vi "Autonomous Independent.vi"() -> ()   [LabVIEW 2014]
doc: "This VI is called when autonomous begins, and will automatically be terminated when autonomous ends. You can carry out timed or sensor driven robot movement independently without needing to return to the caller."
uses:
  <vilib>/Rock Robotics/WPI/Joystick/WPI_JoystickGetSetRefNum.vi
  <vilib>/Rock Robotics/Network Tables/SD Read Boolean.vi
  <vilib>/Rock Robotics/WPI/RobotDrive/WPI_RobotDriveGetSetRefNum.vi
  <vilib>/Rock Robotics/WPI/RobotDrive/WPI_RobotDriveArcadeDrive_Standard(NoSaturation).vi
  <vilib>/Rock Robotics/Network Tables/SD Write Boolean.vi
panel:
  out "Sample Boolean 2":bool
  out "Sample Boolean 3":bool
  out "Sample Boolean 1":bool
  out "Sample Boolean 0":bool
  out "Current Movement, for debugging":T1 {"Y Joystick Value" scale=1.0..-1.0; "X Joystick Value" scale=-1.0..1.0}
  in  "Array of robot movements":T2(array[cluster]) {"Y Joystick Value" scale=1.0..-1.0; "X Joystick Value" scale=-1.0..1.0}
  # "Be sure to right-click and choose Data Operations>>Make Current Value default if you want to save the array values with the VI"
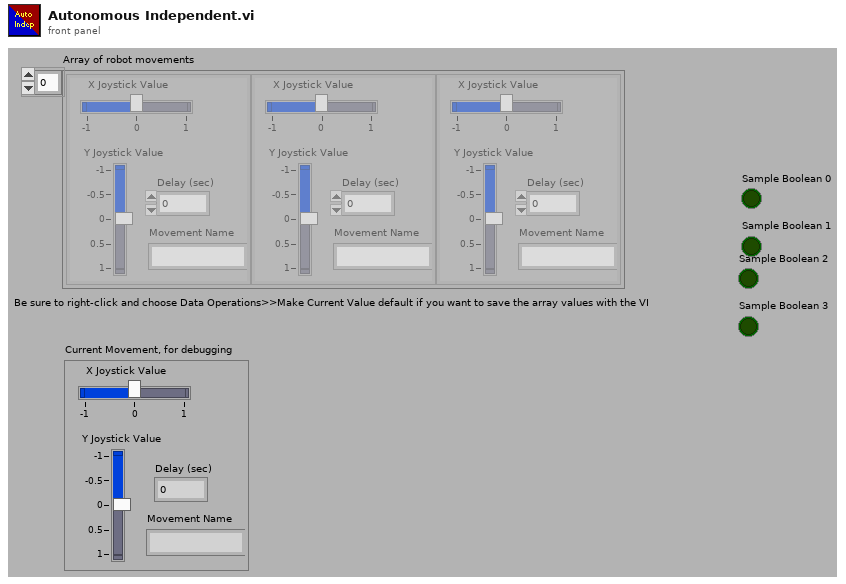
[diagram p1: front panel]
types:
  T1 = cluster{"X Joystick Value":dbl, "Y Joystick Value":dbl, "Delay (sec)":dbl, "Movement Name":string}
  T2 = cluster{"X Joystick Value":dbl, "Y Joystick Value":dbl, "Delay (sec)":dbl, "Movement Name":string}[]
  T3 = typedef "WPI_JoystickDevRef.ctl" = cluster{"Device":T4}
  T4 = typedef "WPI_JoystickDeviceEnum.ctl" = enum16{"USB 0", "USB 1", "USB 2", "USB 3", "USB 4", "USB 5"}
  T5 = typedef "WPI_RobotDriveDevRef.ctl" = cluster{"DevStatus":errorcluster, "Motors[]":T6[], "Square Inputs":bool, "Max Output":dbl}
  T6 = typedef "WPI_MotorControlDeviceRef.ctl" = cluster{"DeviceStatus":errorcluster, "Type":T7, "PWM":cluster{"Controller":T8, "PWM Channel":T9, "DeadBand":T10}, "CAN":cluster{"Device Number":u8, "Control Mode":T11, "Semaphore":T12, "Max Vout":dbl, "TalonSRX Control Mode":T13}, "Invert":bool, "TransformRef":T14, "InvTransformRef":T14}
  T7 = typedef "WPI_MotorControlType.ctl" = enum16{"PWM", "CAN", "CANTalonSRX"}
  T8 = typedef "FPGA_TypedefDigitalModule.ctl" = enum16{"Controller 1"}
  T9 = typedef "FPGA_DIOPWMChannel.ctl" = enum8{"PWM 0", "PWM 1", "PWM 2", "PWM 3", "PWM 4", "PWM 5", "PWM 6", "PWM 7", "PWM 8", "PWM 9", "PWM MXP 0", "PWM MXP 1", "PWM MXP 2", "PWM MXP 3", "PWM MXP 4", "PWM MXP 5", "PWM MXP 6", "PWM MXP 7", "PWM MXP 8", "PWM MXP 9", "Invalid"}
  T10 = typedef "WPI_PWMDeadband.ctl" = cluster{"Name":string, "maxPositivePwm":i32, "minPositivePwm":i32, "centerPwm":i32, "maxNegativePwm":i32, "minNegativePwm":i32, "angularRange":u16}
  T11 = typedef "WPI_CANJaguar_ControlMode.ctl" = enum8{"Percent VBus", "Current", "Speed", "Position", "Voltage"}
  T12 = typedef "Semaphore RefNum" = refnum<k1>
  T13 = typedef "WPI_CANTalonSRX_APIControlMode.ctl" = enum8{"Percent VBus", "Speed", "Position", "Slave", "Unchanged / Invalid"}
  T14 = typedef "WPI_PWMTransform_ConPane.ctl" = refnum<vi>
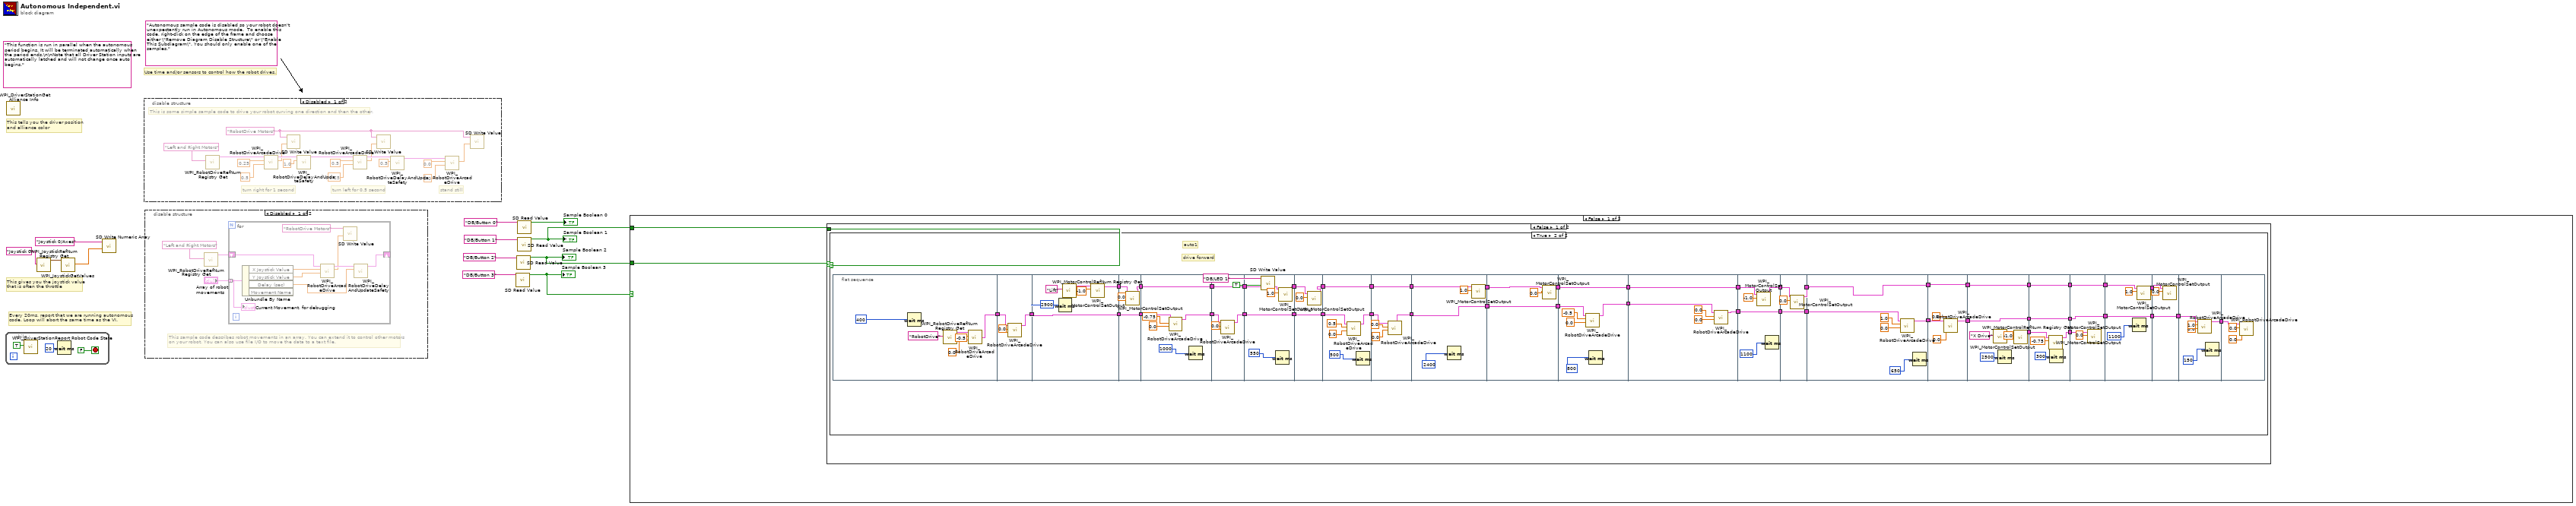
[diagram p0: block diagram]
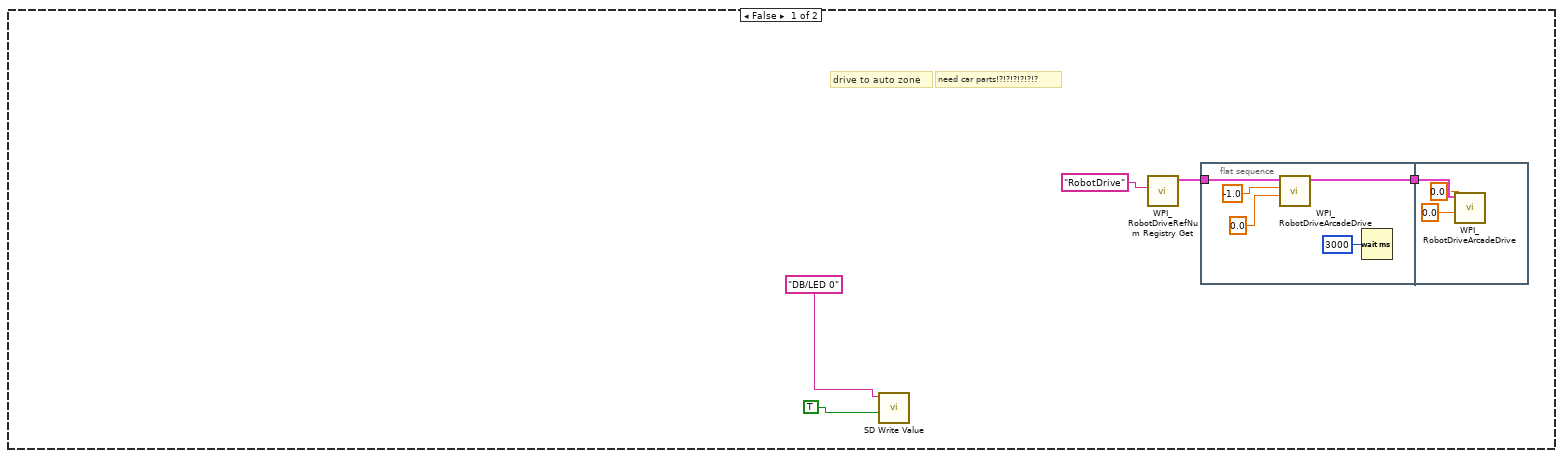
[diagram p2: hidden frame]
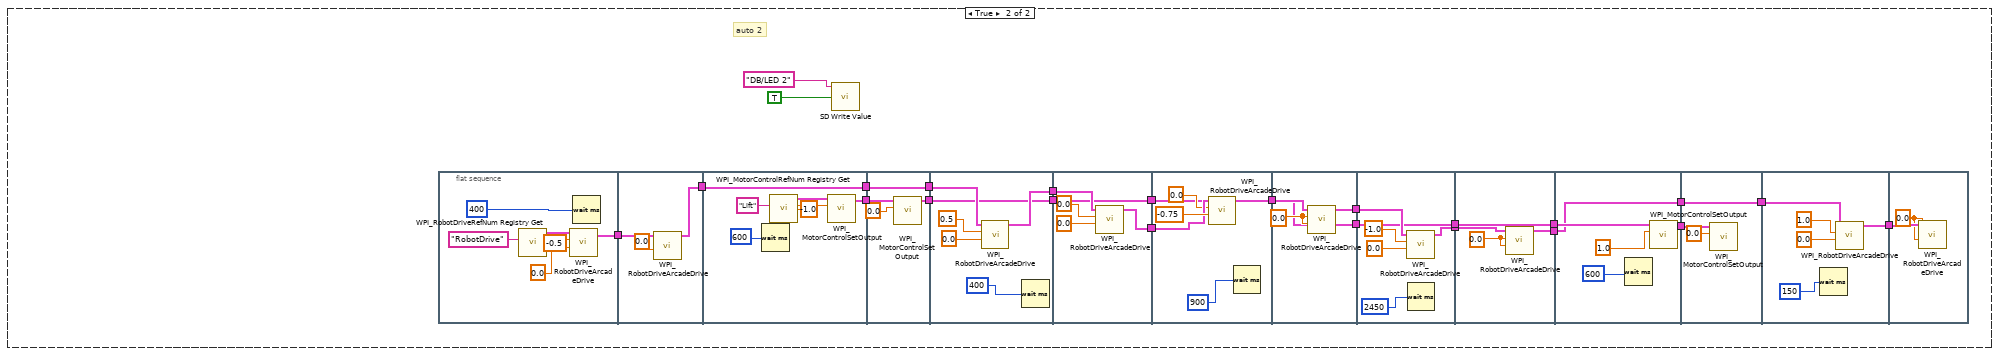
[diagram p3: hidden frame]
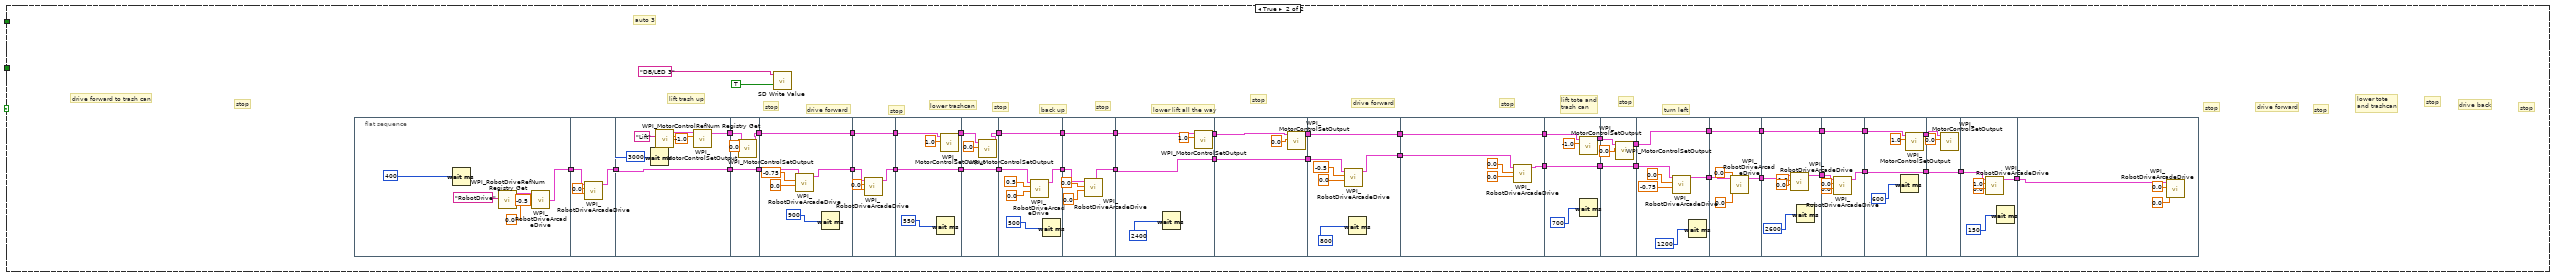
[diagram p4: hidden frame]
diagram:
  (unwired) "Autonomous sample code is disabled so your robot doesn't unexpectantly run in Autonomous mode.  To enable this code, right-click on the edge of the frame and choose either \"Remove Diagram Disable Structure\" or \"Enable This Subdiagram\". You should only enable one of the samples."
  (unwired) "This function is run in parallel when the autonomous period begins. It will be terminated automatically when the period ends.\n\nNote that all Driver Station inputs are automatically latched and will not change once auto begins."
  # "Every 20ms, report that we are running autonomous\ncode. Loop will abort the same time as the VI."
  # "This gives you the joystick value\nthat is often the throttle"
  # "Use time and/or sensors to control how the robot drives."
  # "This tells you the driver position\nand alliance color"
  n1 = while {
    stop <- FALSE stop-if-true
    n2 = call <vilib>:"WPI_DriverStationReport Robot Code State.vi"("Autonomous"=TRUE) -> ()  [unwired: 10 in, 1 out]
    n3 = Wait (ms)(milliseconds to wait=u32 20) -> ()  [unwired: 1 out]
  }
  n4 = call <vilib>:"WPI_DriverStationGet Alliance Info.vi"() -> ()  [unwired: 12 out]
  n5 = call <vilib>:"WPI_JoystickRefNum Registry Get.vi"("refnum name"="Joystick 0") -> ("JoystickDevRef"=w11:T3)  [unwired: 1 in, 9 out]
  n6 = call <vilib>:"WPI_JoystickGetValues.vi"("JoystickDevRef"=w11) -> ("Axes"=w9:dbl[])  [unwired: 6 in, 4 out]
  n7 = call <vilib>:"SD Write Numeric Array.vi"("Numeric Array"=w9, "Name"="Joystick 0/Axes") -> ()  [unwired: 8 in, 2 out]
  n8 = disable-structure shown="Disabled" {
    frame Disabled {
      w19 = "RobotDrive Motors" ("Name")
      # "This is some simple sample code to drive your robot curving one direction and then the other."
      # "stand still"
      # "turn left for 0.5 second"
      # "turn right for 1 second"
      n9 = call <vilib>:"WPI_RobotDriveRefNum Registry Get.vi"("refnum name"="Left and Right Motors") -> ("RobotDriveDevRef"=w20:T5)  [unwired: 1 in, 9 out]
      n10 = call-poly <vilib>:"WPI_RobotDriveArcadeDrive.vi"("Y axis value"=0.5 ("X axis value"), "X axis value"=0.25, "RobotDriveDevRef"=w20) -> ("Motor Values"=w18:dbl[], "RobotDriveDevRef"=w27:T5)  [unwired: 1 in, 6 out]
      n11 = call-poly <vilib>:"SD Write Value.vi"("Numeric Array"=w18, "Name"=w19) -> ()  [unwired: 8 in, 2 out]
      n12 = call <vilib>:"WPI_RobotDriveDelayAndUpdateSafety.vi"("Delay (s)"=1.0, "RobotDriveDevRef"=w27) -> ("RobotDriveDevRef 2"=w26:T5)  [unwired: 8 in, 1 out]
      n13 = call-poly <vilib>:"WPI_RobotDriveArcadeDrive.vi"("Y axis value"=0.25 ("X axis value"), "X axis value"=0.5, "RobotDriveDevRef"=w26) -> ("Motor Values"=w17:dbl[], "RobotDriveDevRef"=w25:T5)  [unwired: 1 in, 6 out]
      n14 = call-poly <vilib>:"SD Write Value.vi"("Numeric Array"=w17, "Name"=w19) -> ()  [unwired: 8 in, 2 out]
      n15 = call <vilib>:"WPI_RobotDriveDelayAndUpdateSafety.vi"("Delay (s)"=0.5, "RobotDriveDevRef"=w25) -> ("RobotDriveDevRef 2"=w24:T5)  [unwired: 8 in, 1 out]
      n16 = call-poly <vilib>:"WPI_RobotDriveArcadeDrive.vi"("Y axis value"=0.0 ("X axis value"), "X axis value"=0.0, "RobotDriveDevRef"=w24) -> ("Motor Values"=w16:dbl[])  [unwired: 1 in, 7 out]
      n17 = call-poly <vilib>:"SD Write Value.vi"("Numeric Array"=w16, "Name"=w19) -> ()  [unwired: 8 in, 2 out]
    }
    frame Enabled {
    }
  }
  n18 = disable-structure shown="Disabled" {
    frame Disabled {
      # "This sample code describes robot movements in an array. You can extend it to control other motors\non your robot. You can also use file I/O to move the data to a text file."
      n19 = call <vilib>:"WPI_RobotDriveRefNum Registry Get.vi"("refnum name"="Left and Right Motors") -> ("RobotDriveDevRef"=w35:T5)  [unwired: 1 in, 9 out]
      n20 = for {
        shift-right: [w42] -> _
        shift-left: w35 -> [w43]
        tunnel: "Array of robot movements" -> [w38] mode=indexing
        n21 = Unbundle By Name(w38) -> ("X Joystick Value"=w41:dbl, "Y Joystick Value"=w40:dbl, "Delay (sec)"=w39:dbl)  [unwired: 1 out]
        n22 = call-poly <vilib>:"WPI_RobotDriveArcadeDrive.vi"("Y axis value"=w40, "X axis value"=w41, "RobotDriveDevRef"=w43) -> ("Motor Values"=w37:dbl[], "RobotDriveDevRef"=w44:T5)  [unwired: 1 in, 6 out]
        n23 = call-poly <vilib>:"SD Write Value.vi"("Numeric Array"=w37, "Name"="RobotDrive Motors") -> ()  [unwired: 8 in, 2 out]
        n24 = call <vilib>:"WPI_RobotDriveDelayAndUpdateSafety.vi"("Delay (s)"=w39, "RobotDriveDevRef"=w44) -> ("RobotDriveDevRef 2"=w42:T5)  [unwired: 8 in, 1 out]
        "Current Movement, for debugging" <- w38
      }
    }
    frame Enabled {
    }
  }
  n25 = call-poly <vilib>:"SD Read Value.vi"("Name"="DB/Button 3" ("refnum name")) -> ("Boolean"=w3:bool)  [unwired: 8 in, 2 out]
  "Sample Boolean 3" <- w3
  n26 = call-poly <vilib>:"SD Read Value.vi"("Name"="DB/Button 2" ("refnum name")) -> ("Boolean"=w2:bool)  [unwired: 8 in, 2 out]
  "Sample Boolean 2" <- w2
  n27 = call-poly <vilib>:"SD Read Value.vi"("Name"="DB/Button 1" ("refnum name")) -> ("Boolean"=w1:bool)  [unwired: 8 in, 2 out]
  "Sample Boolean 1" <- w1
  n28 = call-poly <vilib>:"SD Read Value.vi"("Name"="DB/Button 0" ("refnum name")) -> ("Boolean"=→"Sample Boolean 0":bool)  [unwired: 8 in, 2 out]
  n29 = case shown="False" w3 {
    tunnel: w2 -> [w47 _]
    tunnel: w1 -> [w46 _]
    frame False {
      n30 = case shown="False" w47 {
        tunnel: w46 -> [w48 _]
        frame False {
          n31 = case shown="True" w48 {
            frame False {
              # "need car parts!?!?!?!?!?!?"
              # "drive to auto zone"
              n32 = call-poly <vilib>:"SD Write Value.vi"("Boolean"=TRUE, "Name"="DB/LED 0" ("refnum name")) -> ()  [unwired: 8 in, 2 out]
              n33 = call <vilib>:"WPI_RobotDriveRefNum Registry Get.vi"("refnum name"="RobotDrive") -> ("RobotDriveDevRef"=w53:T5)  [unwired: 1 in, 9 out]
              n34 = flat-sequence {
                tunnel: w53 -> [w56]
                tunnel: [w54] -> w49
                tunnel: w49 -> [w61]
                frame #0 {
                  n35 = call-poly <vilib>:"WPI_RobotDriveArcadeDrive.vi"("Y axis value"=0.0 ("X axis value"), "X axis value"=-1.0, "RobotDriveDevRef"=w56) -> ("RobotDriveDevRef"=w54:T5)  [unwired: 1 in, 7 out]
                  n36 = Wait (ms)(milliseconds to wait=u32 3000) -> ()  [unwired: 1 out]
                }
                frame #1 {
                  n37 = call-poly <vilib>:"WPI_RobotDriveArcadeDrive.vi"("Y axis value"=0.0, "X axis value"=0.0, "RobotDriveDevRef"=w61) -> ()  [unwired: 1 in, 8 out]
                }
              }
            }
            frame True {
              # "drive forward"
              # "auto1"
              n38 = flat-sequence {
                tunnel: [w111] -> w107
                tunnel: w107 -> [w118]
                tunnel: [w117] -> w106
                tunnel: w106 -> [w121]
                tunnel: [w121] -> w105
                tunnel: [w119] -> w104
                tunnel: w105 -> [w128]
                tunnel: [w128] -> w103
                tunnel: w104 -> [w127]
                tunnel: [w126] -> w102
                tunnel: w103 -> [w132]
                tunnel: [w131] -> w101
                tunnel: w102 -> [w129]
                tunnel: [w129] -> w100
                tunnel: w101 -> [w137]
                tunnel: [w136] -> w99
                tunnel: w100 -> [w138]
                tunnel: [w138] -> w98
                tunnel: w99 -> [w143]
                tunnel: [w143] -> w97
                tunnel: w98 -> [w141]
                tunnel: [w140] -> w96
                tunnel: w97 -> [w147]
                tunnel: [w147] -> w95
                tunnel: w96 -> [w145]
                tunnel: [w144] -> w94
                tunnel: w95 -> [w152]
                tunnel: [w151] -> w93
                tunnel: w94 -> [w153]
                tunnel: [w153] -> w92
                tunnel: w93 -> [w157]
                tunnel: [w156] -> w91
                tunnel: w92 -> [w158]
                tunnel: [w158] -> w90
                tunnel: w91 -> [w162]
                tunnel: [w162] -> w89
                tunnel: [w161] -> w88
                tunnel: w90 -> [w160]
                tunnel: w89 -> [w167]
                tunnel: [w167] -> w87
                tunnel: w88 -> [w165]
                tunnel: [w164] -> w86
                tunnel: w87 -> [w171]
                tunnel: [w170] -> w85
                tunnel: w86 -> [w168]
                tunnel: [w168] -> w84
                tunnel: w85 -> [w176]
                tunnel: w84 -> [w175]
                tunnel: [w175] -> w73
                tunnel: [w174] -> w72
                tunnel: w73 -> [w181]
                tunnel: [w180] -> w71
                tunnel: w72 -> [w183]
                tunnel: [w183] -> w69
                tunnel: w71 -> [w186]
                tunnel: [w185] -> w70
                tunnel: w69 -> [w187]
                tunnel: [w187] -> w68
                tunnel: [w189] -> w83
                tunnel: [w188] -> w82
                tunnel: w70 -> [w188]
                tunnel: w68 -> [w191]
                tunnel: w83 -> [w198]
                tunnel: [w195] -> w81
                tunnel: w82 -> [w194]
                tunnel: [w194] -> w80
                tunnel: w81 -> [w204]
                tunnel: w80 -> [w205]
                tunnel: [w205] -> w67
                tunnel: [w204] -> w65
                tunnel: [w200] -> w63
                tunnel: w67 -> [w211]
                tunnel: [w211] -> w66
                tunnel: w65 -> [w210]
                tunnel: [w210] -> w64
                tunnel: w63 -> [w208]
                tunnel: [w209] -> w62
                tunnel: w66 -> [w215]
                tunnel: [w215] -> w79
                tunnel: [w214] -> w78
                tunnel: w64 -> [w214]
                tunnel: w62 -> [w213]
                tunnel: [w219] -> w77
                tunnel: w79 -> [w218]
                tunnel: [w216] -> w76
                tunnel: w78 -> [w216]
                tunnel: w77 -> [w222]
                tunnel: [w221] -> w75
                tunnel: w76 -> [w221]
                tunnel: w75 -> [w228]
                tunnel: [w224] -> w74
                tunnel: w74 -> [w231]
                frame #0 {
                  n39 = Wait (ms)(milliseconds to wait=u32 400) -> ()  [unwired: 1 out]
                  n40 = call <vilib>:"WPI_RobotDriveRefNum Registry Get.vi"("refnum name"="RobotDrive") -> ("RobotDriveDevRef"=w114:T5)  [unwired: 1 in, 9 out]
                  n41 = call-poly <vilib>:"WPI_RobotDriveArcadeDrive.vi"("Y axis value"=0.0 ("X axis value"), "X axis value"=-0.5, "RobotDriveDevRef"=w114) -> ("RobotDriveDevRef"=w111:T5)  [unwired: 1 in, 7 out]
                }
                frame #1 {
                  w116 = 0.0 ("X axis value")
                  n42 = call-poly <vilib>:"WPI_RobotDriveArcadeDrive.vi"("Y axis value"=w116, "X axis value"=w116, "RobotDriveDevRef"=w118) -> ("RobotDriveDevRef"=w117:T5)  [unwired: 1 in, 7 out]
                }
                frame #2 {
                  n43 = Wait (ms)(milliseconds to wait=u32 2900) -> ()  [unwired: 1 out]
                  n44 = call <vilib>:"WPI_MotorControlRefNum Registry Get.vi"("refnum name"="Lift") -> ("MotorControlDevRef"=w123:T6)  [unwired: 9 in, 1 out]
                  n45 = call <vilib>:"WPI_MotorControlSetOutput.vi"("Output"=-1.0, "MotorControlDevRef"=w123) -> ("MotorControlDevRef"=w119:T6)  [unwired: 7 in, 2 out]
                }
                frame #3 {
                  n46 = call <vilib>:"WPI_MotorControlSetOutput.vi"("Output"=0.0, "MotorControlDevRef"=w127) -> ("MotorControlDevRef"=w126:T6)  [unwired: 7 in, 2 out]
                }
                frame #4 {
                  n47 = call-poly <vilib>:"WPI_RobotDriveArcadeDrive.vi"("Y axis value"=0.0 ("X axis value"), "X axis value"=-0.75, "RobotDriveDevRef"=w132) -> ("RobotDriveDevRef"=w131:T5)  [unwired: 1 in, 7 out]
                  n48 = Wait (ms)(milliseconds to wait=u32 1000) -> ()  [unwired: 1 out]
                }
                frame #5 {
                  w135 = 0.0 ("X axis value")
                  n49 = call-poly <vilib>:"WPI_RobotDriveArcadeDrive.vi"("Y axis value"=w135, "X axis value"=w135, "RobotDriveDevRef"=w137) -> ("RobotDriveDevRef"=w136:T5)  [unwired: 1 in, 7 out]
                }
                frame #6 {
                  n50 = Wait (ms)(milliseconds to wait=u32 550) -> ()  [unwired: 1 out]
                  n51 = call <vilib>:"WPI_MotorControlSetOutput.vi"("Output"=1.0, "MotorControlDevRef"=w141) -> ("MotorControlDevRef"=w140:T6)  [unwired: 7 in, 2 out]
                }
                frame #7 {
                  n52 = call <vilib>:"WPI_MotorControlSetOutput.vi"("Output"=0.0, "MotorControlDevRef"=w145) -> ("MotorControlDevRef"=w144:T6)  [unwired: 7 in, 2 out]
                }
                frame #8 {
                  n53 = call-poly <vilib>:"WPI_RobotDriveArcadeDrive.vi"("Y axis value"=0.0, "X axis value"=0.5, "RobotDriveDevRef"=w152) -> ("RobotDriveDevRef"=w151:T5)  [unwired: 1 in, 7 out]
                  n54 = Wait (ms)(milliseconds to wait=u32 500) -> ()  [unwired: 1 out]
                }
                frame #9 {
                  n55 = call-poly <vilib>:"WPI_RobotDriveArcadeDrive.vi"("Y axis value"=0.0, "X axis value"=0.0, "RobotDriveDevRef"=w157) -> ("RobotDriveDevRef"=w156:T5)  [unwired: 1 in, 7 out]
                }
                frame #10 {
                  n56 = Wait (ms)(milliseconds to wait=u32 2400) -> ()  [unwired: 1 out]
                  n57 = call <vilib>:"WPI_MotorControlSetOutput.vi"("Output"=1.0, "MotorControlDevRef"=w160) -> ("MotorControlDevRef"=w161:T6)  [unwired: 7 in, 2 out]
                }
                frame #11 {
                  n58 = call <vilib>:"WPI_MotorControlSetOutput.vi"("Output"=0.0, "MotorControlDevRef"=w165) -> ("MotorControlDevRef"=w164:T6)  [unwired: 7 in, 2 out]
                }
                frame #12 {
                  n59 = call-poly <vilib>:"WPI_RobotDriveArcadeDrive.vi"("Y axis value"=0.0 ("X axis value"), "X axis value"=-0.5, "RobotDriveDevRef"=w171) -> ("RobotDriveDevRef"=w170:T5)  [unwired: 1 in, 7 out]
                  n60 = Wait (ms)(milliseconds to wait=u32 800) -> ()  [unwired: 1 out]
                }
                frame #13 {
                  n61 = call-poly <vilib>:"WPI_RobotDriveArcadeDrive.vi"("Y axis value"=0.0 ("X axis value"), "X axis value"=0.0, "RobotDriveDevRef"=w176) -> ("RobotDriveDevRef"=w174:T5)  [unwired: 1 in, 7 out]
                }
                frame #14 {
                  n62 = call <vilib>:"WPI_MotorControlSetOutput.vi"("Output"=-1.0, "MotorControlDevRef"=w181) -> ("MotorControlDevRef"=w180:T6)  [unwired: 7 in, 2 out]
                  n63 = Wait (ms)(milliseconds to wait=u32 1100) -> ()  [unwired: 1 out]
                }
                frame #15 {
                  n64 = call <vilib>:"WPI_MotorControlSetOutput.vi"("Output"=0.0, "MotorControlDevRef"=w186) -> ("MotorControlDevRef"=w185:T6)  [unwired: 7 in, 2 out]
                }
                frame #16 {
                  n65 = call-poly <vilib>:"WPI_RobotDriveArcadeDrive.vi"("Y axis value"=0.0 ("X axis value"), "X axis value"=1.0, "RobotDriveDevRef"=w191) -> ("RobotDriveDevRef"=w189:T5)  [unwired: 1 in, 7 out]
                  n66 = Wait (ms)(milliseconds to wait=u32 650) -> ()  [unwired: 1 out]
                }
                frame #17 {
                  n67 = call-poly <vilib>:"WPI_RobotDriveArcadeDrive.vi"("Y axis value"=0.0, "X axis value"=0.0, "RobotDriveDevRef"=w198) -> ("RobotDriveDevRef"=w195:T5)  [unwired: 1 in, 7 out]
                }
                frame #18 {
                  n68 = call <vilib>:"WPI_MotorControlRefNum Registry Get.vi"("refnum name"="X Drive") -> ("MotorControlDevRef"=w202:T6)  [unwired: 9 in, 1 out]
                  n69 = Wait (ms)(milliseconds to wait=u32 2500) -> ()  [unwired: 1 out]
                  n70 = call <vilib>:"WPI_MotorControlSetOutput.vi"("Output"=-1.0, "MotorControlDevRef"=w202) -> ("MotorControlDevRef"=w200:T6)  [unwired: 7 in, 2 out]
                }
                frame #19 {
                  n71 = call <vilib>:"WPI_MotorControlSetOutput.vi"("Output"=-0.75, "MotorControlDevRef"=w208) -> ("MotorControlDevRef"=w209:T6)  [unwired: 7 in, 2 out]
                  n72 = Wait (ms)(milliseconds to wait=u32 300) -> ()  [unwired: 1 out]
                }
                frame #20 {
                  n73 = call <vilib>:"WPI_MotorControlSetOutput.vi"("Output"=0.0, "MotorControlDevRef"=w213) -> ()  [unwired: 7 in, 3 out]
                }
                frame #21 {
                  n74 = Wait (ms)(milliseconds to wait=u32 1100) -> ()  [unwired: 1 out]
                  n75 = call <vilib>:"WPI_MotorControlSetOutput.vi"("Output"=1.0, "MotorControlDevRef"=w218) -> ("MotorControlDevRef"=w219:T6)  [unwired: 7 in, 2 out]
                }
                frame #22 {
                  n76 = call <vilib>:"WPI_MotorControlSetOutput.vi"("Output"=0.0, "MotorControlDevRef"=w222) -> ()  [unwired: 7 in, 3 out]
                }
                frame #23 {
                  n77 = call-poly <vilib>:"WPI_RobotDriveArcadeDrive.vi"("Y axis value"=0.0, "X axis value"=1.0, "RobotDriveDevRef"=w228) -> ("RobotDriveDevRef"=w224:T5)  [unwired: 1 in, 7 out]
                  n78 = Wait (ms)(milliseconds to wait=u32 150) -> ()  [unwired: 1 out]
                }
                frame #24 {
                  n79 = call-poly <vilib>:"WPI_RobotDriveArcadeDrive.vi"("Y axis value"=0.0, "X axis value"=0.0, "RobotDriveDevRef"=w231) -> ()  [unwired: 1 in, 8 out]
                }
              }
              n80 = call-poly <vilib>:"SD Write Value.vi"("Boolean"=TRUE, "Name"="DB/LED 1" ("refnum name")) -> ()  [unwired: 8 in, 2 out]
            }
          }
        }
        frame True {
          # "auto 2"
          n81 = flat-sequence {
            tunnel: [w256] -> w253
            tunnel: w253 -> [w263]
            tunnel: [w262] -> w251
            tunnel: [w266] -> w252
            tunnel: w251 -> [w265]
            tunnel: [w265] -> w250
            tunnel: w252 -> [w273]
            tunnel: w250 -> [w272]
            tunnel: [w272] -> w249
            tunnel: [w271] -> w242
            tunnel: w249 -> [w277]
            tunnel: [w276] -> w248
            tunnel: w242 -> [w275]
            tunnel: [w275] -> w241
            tunnel: w248 -> [w284]
            tunnel: [w282] -> w247
            tunnel: w241 -> [w281]
            tunnel: [w281] -> w240
            tunnel: w247 -> [w289]
            tunnel: [w287] -> w246
            tunnel: w240 -> [w286]
            tunnel: [w286] -> w239
            tunnel: w246 -> [w294]
            tunnel: [w293] -> w245
            tunnel: w239 -> [w292]
            tunnel: [w292] -> w238
            tunnel: w245 -> [w300]
            tunnel: [w297] -> w244
            tunnel: w238 -> [w296]
            tunnel: [w296] -> w237
            tunnel: w244 -> [w304]
            tunnel: [w303] -> w243
            tunnel: w237 -> [w302]
            tunnel: [w302] -> w236
            tunnel: w243 -> [w306]
            tunnel: w236 -> [w308]
            tunnel: [w307] -> w235
            tunnel: [w306] -> w234
            tunnel: w235 -> [w313]
            tunnel: w234 -> [w311]
            tunnel: [w311] -> w233
            tunnel: w233 -> [w316]
            tunnel: [w314] -> w232
            tunnel: w232 -> [w320]
            frame #0 {
              n82 = call <vilib>:"WPI_RobotDriveRefNum Registry Get.vi"("refnum name"="RobotDrive") -> ("RobotDriveDevRef"=w260:T5)  [unwired: 1 in, 9 out]
              n83 = call-poly <vilib>:"WPI_RobotDriveArcadeDrive.vi"("Y axis value"=0.0 ("X axis value"), "X axis value"=-0.5, "RobotDriveDevRef"=w260) -> ("RobotDriveDevRef"=w256:T5)  [unwired: 1 in, 7 out]
              n84 = Wait (ms)(milliseconds to wait=u32 400) -> ()  [unwired: 1 out]
            }
            frame #1 {
              n85 = call-poly <vilib>:"WPI_RobotDriveArcadeDrive.vi"("Y axis value"=0.0 ("X axis value"), "RobotDriveDevRef"=w263) -> ("RobotDriveDevRef"=w262:T5)  [unwired: 2 in, 7 out]
            }
            frame #2 {
              n86 = Wait (ms)(milliseconds to wait=u32 600) -> ()  [unwired: 1 out]
              n87 = call <vilib>:"WPI_MotorControlRefNum Registry Get.vi"("refnum name"="Lift") -> ("MotorControlDevRef"=w268:T6)  [unwired: 9 in, 1 out]
              n88 = call <vilib>:"WPI_MotorControlSetOutput.vi"("Output"=-1.0, "MotorControlDevRef"=w268) -> ("MotorControlDevRef"=w266:T6)  [unwired: 7 in, 2 out]
            }
            frame #3 {
              n89 = call <vilib>:"WPI_MotorControlSetOutput.vi"("Output"=0.0, "MotorControlDevRef"=w273) -> ("MotorControlDevRef"=w271:T6)  [unwired: 7 in, 2 out]
            }
            frame #4 {
              n90 = call-poly <vilib>:"WPI_RobotDriveArcadeDrive.vi"("Y axis value"=0.0 ("X axis value"), "X axis value"=0.5, "RobotDriveDevRef"=w277) -> ("RobotDriveDevRef"=w276:T5)  [unwired: 1 in, 7 out]
              n91 = Wait (ms)(milliseconds to wait=u32 400) -> ()  [unwired: 1 out]
            }
            frame #5 {
              n92 = call-poly <vilib>:"WPI_RobotDriveArcadeDrive.vi"("Y axis value"=0.0 ("X axis value"), "X axis value"=0.0, "RobotDriveDevRef"=w284) -> ("RobotDriveDevRef"=w282:T5)  [unwired: 1 in, 7 out]
            }
            frame #6 {
              n93 = call-poly <vilib>:"WPI_RobotDriveArcadeDrive.vi"("Y axis value"=-0.75 ("X axis value"), "X axis value"=0.0, "RobotDriveDevRef"=w289) -> ("RobotDriveDevRef"=w287:T5)  [unwired: 1 in, 7 out]
              n94 = Wait (ms)(milliseconds to wait=u32 900) -> ()  [unwired: 1 out]
            }
            frame #7 {
              w295 = 0.0 ("X axis value")
              n95 = call-poly <vilib>:"WPI_RobotDriveArcadeDrive.vi"("Y axis value"=w295, "X axis value"=w295, "RobotDriveDevRef"=w294) -> ("RobotDriveDevRef"=w293:T5)  [unwired: 1 in, 7 out]
            }
            frame #8 {
              n96 = call-poly <vilib>:"WPI_RobotDriveArcadeDrive.vi"("Y axis value"=0.0 ("X axis value"), "X axis value"=-1.0, "RobotDriveDevRef"=w300) -> ("RobotDriveDevRef"=w297:T5)  [unwired: 1 in, 7 out]
              n97 = Wait (ms)(milliseconds to wait=u32 2450) -> ()  [unwired: 1 out]
            }
            frame #9 {
              w305 = 0.0 ("X axis value")
              n98 = call-poly <vilib>:"WPI_RobotDriveArcadeDrive.vi"("Y axis value"=w305, "X axis value"=w305, "RobotDriveDevRef"=w304) -> ("RobotDriveDevRef"=w303:T5)  [unwired: 1 in, 7 out]
            }
            frame #10 {
              n99 = Wait (ms)(milliseconds to wait=u32 600) -> ()  [unwired: 1 out]
              n100 = call <vilib>:"WPI_MotorControlSetOutput.vi"("Output"=1.0, "MotorControlDevRef"=w308) -> ("MotorControlDevRef"=w307:T6)  [unwired: 7 in, 2 out]
            }
            frame #11 {
              n101 = call <vilib>:"WPI_MotorControlSetOutput.vi"("Output"=0.0, "MotorControlDevRef"=w313) -> ()  [unwired: 7 in, 3 out]
            }
            frame #12 {
              n102 = Wait (ms)(milliseconds to wait=u32 150) -> ()  [unwired: 1 out]
              n103 = call-poly <vilib>:"WPI_RobotDriveArcadeDrive.vi"("Y axis value"=0.0 ("X axis value"), "X axis value"=1.0, "RobotDriveDevRef"=w316) -> ("RobotDriveDevRef"=w314:T5)  [unwired: 1 in, 7 out]
            }
            frame #13 {
              w319 = 0.0 ("X axis value")
              n104 = call-poly <vilib>:"WPI_RobotDriveArcadeDrive.vi"("Y axis value"=w319, "X axis value"=w319, "RobotDriveDevRef"=w320) -> ()  [unwired: 1 in, 8 out]
            }
          }
          n105 = call-poly <vilib>:"SD Write Value.vi"("Boolean"=TRUE, "Name"="DB/LED 2" ("refnum name")) -> ()  [unwired: 8 in, 2 out]
        }
      }
    }
    frame True {
      # "stop"
      # "drive back"
      # "stop"
      # "lower tote \nand trashcan"
      # "stop"
      # "drive forward"
      # "stop"
      # "turn left"
      # "stop"
      # "lift tote and\ntrash can"
      # "stop"
      # "drive forward"
      # "stop"
      # "lower lift all the way"
      # "stop"
      # "back up"
      # "stop"
      # "lower trashcan"
      # "stop"
      # "drive forward"
      # "stop"
      # "lift trash up"
      # "stop"
      # "drive forward to trash can"
      # "auto 3"
      n106 = flat-sequence {
        tunnel: [w366] -> w359
        tunnel: w359 -> [w373]
        tunnel: [w372] -> w358
        tunnel: w358 -> [w376]
        tunnel: [w376] -> w356
        tunnel: [w374] -> w354
        tunnel: w356 -> [w383]
        tunnel: [w383] -> w355
        tunnel: w354 -> [w382]
        tunnel: [w381] -> w353
        tunnel: w355 -> [w387]
        tunnel: [w386] -> w352
        tunnel: w353 -> [w384]
        tunnel: [w384] -> w351
        tunnel: w352 -> [w392]
        tunnel: [w391] -> w346
        tunnel: w351 -> [w393]
        tunnel: [w393] -> w345
        tunnel: w346 -> [w398]
        tunnel: [w398] -> w344
        tunnel: w345 -> [w396]
        tunnel: [w395] -> w342
        tunnel: w344 -> [w402]
        tunnel: [w402] -> w343
        tunnel: w342 -> [w400]
        tunnel: [w399] -> w341
        tunnel: w343 -> [w407]
        tunnel: [w406] -> w350
        tunnel: w341 -> [w408]
        tunnel: [w408] -> w348
        tunnel: w350 -> [w412]
        tunnel: [w411] -> w349
        tunnel: w348 -> [w413]
        tunnel: [w413] -> w347
        tunnel: w349 -> [w417]
        tunnel: [w417] -> w361
        tunnel: [w416] -> w357
        tunnel: w347 -> [w415]
        tunnel: w361 -> [w422]
        tunnel: [w422] -> w360
        tunnel: w357 -> [w420]
        tunnel: [w419] -> w340
        tunnel: w360 -> [w426]
        tunnel: [w425] -> w362
        tunnel: w340 -> [w423]
        tunnel: [w423] -> w339
        tunnel: w362 -> [w431]
        tunnel: w339 -> [w430]
        tunnel: [w430] -> w338
        tunnel: [w429] -> w336
        tunnel: w338 -> [w438]
        tunnel: [w436] -> w337
        tunnel: w336 -> [w435]
        tunnel: [w435] -> w335
        tunnel: w337 -> [w441]
        tunnel: w335 -> [w440]
        tunnel: [w440] -> w334
        tunnel: [w439] -> w329
        tunnel: w334 -> [w446]
        tunnel: [w444] -> w333
        tunnel: w329 -> [w443]
        tunnel: [w443] -> w328
        tunnel: w333 -> [w453]
        tunnel: [w450] -> w331
        tunnel: w328 -> [w449]
        tunnel: [w449] -> w327
        tunnel: [w459] -> w332
        tunnel: w331 -> [w458]
        tunnel: w327 -> [w454]
        tunnel: [w454] -> w326
        tunnel: w332 -> [w464]
        tunnel: w326 -> [w461]
        tunnel: [w461] -> w325
        tunnel: [w460] -> w322
        tunnel: [w468] -> w330
        tunnel: w325 -> [w467]
        tunnel: [w465] -> w323
        tunnel: w322 -> [w465]
        tunnel: w330 -> [w471]
        tunnel: [w470] -> w324
        tunnel: w323 -> [w470]
        tunnel: w324 -> [w477]
        tunnel: [w473] -> w321
        tunnel: w321 -> [w480]
        frame #0 {
          n107 = Wait (ms)(milliseconds to wait=u32 400) -> ()  [unwired: 1 out]
          n108 = call <vilib>:"WPI_RobotDriveRefNum Registry Get.vi"("refnum name"="RobotDrive") -> ("RobotDriveDevRef"=w369:T5)  [unwired: 1 in, 9 out]
          n109 = call-poly <vilib>:"WPI_RobotDriveArcadeDrive.vi"("Y axis value"=0.0 ("X axis value"), "X axis value"=-0.5, "RobotDriveDevRef"=w369) -> ("RobotDriveDevRef"=w366:T5)  [unwired: 1 in, 7 out]
        }
        frame #1 {
          w371 = 0.0 ("X axis value")
          n110 = call-poly <vilib>:"WPI_RobotDriveArcadeDrive.vi"("Y axis value"=w371, "X axis value"=w371, "RobotDriveDevRef"=w373) -> ("RobotDriveDevRef"=w372:T5)  [unwired: 1 in, 7 out]
        }
        frame #2 {
          n111 = Wait (ms)(milliseconds to wait=u32 3000) -> ()  [unwired: 1 out]
          n112 = call <vilib>:"WPI_MotorControlRefNum Registry Get.vi"("refnum name"="Lift") -> ("MotorControlDevRef"=w378:T6)  [unwired: 9 in, 1 out]
          n113 = call <vilib>:"WPI_MotorControlSetOutput.vi"("Output"=-1.0, "MotorControlDevRef"=w378) -> ("MotorControlDevRef"=w374:T6)  [unwired: 7 in, 2 out]
        }
        frame #3 {
          n114 = call <vilib>:"WPI_MotorControlSetOutput.vi"("Output"=0.0, "MotorControlDevRef"=w382) -> ("MotorControlDevRef"=w381:T6)  [unwired: 7 in, 2 out]
        }
        frame #4 {
          n115 = call-poly <vilib>:"WPI_RobotDriveArcadeDrive.vi"("Y axis value"=0.0 ("X axis value"), "X axis value"=-0.75, "RobotDriveDevRef"=w387) -> ("RobotDriveDevRef"=w386:T5)  [unwired: 1 in, 7 out]
          n116 = Wait (ms)(milliseconds to wait=u32 900) -> ()  [unwired: 1 out]
        }
        frame #5 {
          w390 = 0.0 ("X axis value")
          n117 = call-poly <vilib>:"WPI_RobotDriveArcadeDrive.vi"("Y axis value"=w390, "X axis value"=w390, "RobotDriveDevRef"=w392) -> ("RobotDriveDevRef"=w391:T5)  [unwired: 1 in, 7 out]
        }
        frame #6 {
          n118 = Wait (ms)(milliseconds to wait=u32 550) -> ()  [unwired: 1 out]
          n119 = call <vilib>:"WPI_MotorControlSetOutput.vi"("Output"=1.0, "MotorControlDevRef"=w396) -> ("MotorControlDevRef"=w395:T6)  [unwired: 7 in, 2 out]
        }
        frame #7 {
          n120 = call <vilib>:"WPI_MotorControlSetOutput.vi"("Output"=0.0, "MotorControlDevRef"=w400) -> ("MotorControlDevRef"=w399:T6)  [unwired: 7 in, 2 out]
        }
        frame #8 {
          n121 = call-poly <vilib>:"WPI_RobotDriveArcadeDrive.vi"("Y axis value"=0.0, "X axis value"=0.5, "RobotDriveDevRef"=w407) -> ("RobotDriveDevRef"=w406:T5)  [unwired: 1 in, 7 out]
          n122 = Wait (ms)(milliseconds to wait=u32 500) -> ()  [unwired: 1 out]
        }
        frame #9 {
          n123 = call-poly <vilib>:"WPI_RobotDriveArcadeDrive.vi"("Y axis value"=0.0, "X axis value"=0.0, "RobotDriveDevRef"=w412) -> ("RobotDriveDevRef"=w411:T5)  [unwired: 1 in, 7 out]
        }
        frame #10 {
          n124 = Wait (ms)(milliseconds to wait=u32 2400) -> ()  [unwired: 1 out]
          n125 = call <vilib>:"WPI_MotorControlSetOutput.vi"("Output"=1.0, "MotorControlDevRef"=w415) -> ("MotorControlDevRef"=w416:T6)  [unwired: 7 in, 2 out]
        }
        frame #11 {
          n126 = call <vilib>:"WPI_MotorControlSetOutput.vi"("Output"=0.0, "MotorControlDevRef"=w420) -> ("MotorControlDevRef"=w419:T6)  [unwired: 7 in, 2 out]
        }
        frame #12 {
          n127 = call-poly <vilib>:"WPI_RobotDriveArcadeDrive.vi"("Y axis value"=0.0 ("X axis value"), "X axis value"=-0.5, "RobotDriveDevRef"=w426) -> ("RobotDriveDevRef"=w425:T5)  [unwired: 1 in, 7 out]
          n128 = Wait (ms)(milliseconds to wait=u32 800) -> ()  [unwired: 1 out]
        }
        frame #13 {
          n129 = call-poly <vilib>:"WPI_RobotDriveArcadeDrive.vi"("Y axis value"=0.0 ("X axis value"), "X axis value"=0.0, "RobotDriveDevRef"=w431) -> ("RobotDriveDevRef"=w429:T5)  [unwired: 1 in, 7 out]
        }
        frame #14 {
          n130 = call <vilib>:"WPI_MotorControlSetOutput.vi"("Output"=-1.0, "MotorControlDevRef"=w438) -> ("MotorControlDevRef"=w436:T6)  [unwired: 7 in, 2 out]
          n131 = Wait (ms)(milliseconds to wait=u32 700) -> ()  [unwired: 1 out]
        }
        frame #15 {
          n132 = call <vilib>:"WPI_MotorControlSetOutput.vi"("Output"=0.0, "MotorControlDevRef"=w441) -> ("MotorControlDevRef"=w439:T6)  [unwired: 7 in, 2 out]
        }
        frame #16 {
          n133 = call-poly <vilib>:"WPI_RobotDriveArcadeDrive.vi"("Y axis value"=-0.75 ("X axis value"), "X axis value"=0.0, "RobotDriveDevRef"=w446) -> ("RobotDriveDevRef"=w444:T5)  [unwired: 1 in, 7 out]
          n134 = Wait (ms)(milliseconds to wait=u32 1200) -> ()  [unwired: 1 out]
        }
        frame #17 {
          n135 = call-poly <vilib>:"WPI_RobotDriveArcadeDrive.vi"("Y axis value"=0.0, "X axis value"=0.0, "RobotDriveDevRef"=w453) -> ("RobotDriveDevRef"=w450:T5)  [unwired: 1 in, 7 out]
        }
        frame #18 {
          n136 = call-poly <vilib>:"WPI_RobotDriveArcadeDrive.vi"("Y axis value"=0.0, "X axis value"=-1.0, "RobotDriveDevRef"=w458) -> ("RobotDriveDevRef"=w459:T5)  [unwired: 1 in, 7 out]
          n137 = Wait (ms)(milliseconds to wait=u32 2600) -> ()  [unwired: 1 out]
        }
        frame #19 {
          n138 = call-poly <vilib>:"WPI_RobotDriveArcadeDrive.vi"("Y axis value"=0.0, "X axis value"=0.0, "RobotDriveDevRef"=w464) -> ("RobotDriveDevRef"=w460:T5)  [unwired: 1 in, 7 out]
        }
        frame #20 {
          n139 = Wait (ms)(milliseconds to wait=u32 600) -> ()  [unwired: 1 out]
          n140 = call <vilib>:"WPI_MotorControlSetOutput.vi"("Output"=1.0, "MotorControlDevRef"=w467) -> ("MotorControlDevRef"=w468:T6)  [unwired: 7 in, 2 out]
        }
        frame #21 {
          n141 = call <vilib>:"WPI_MotorControlSetOutput.vi"("Output"=0.0, "MotorControlDevRef"=w471) -> ()  [unwired: 7 in, 3 out]
        }
        frame #22 {
          n142 = call-poly <vilib>:"WPI_RobotDriveArcadeDrive.vi"("Y axis value"=0.0, "X axis value"=1.0, "RobotDriveDevRef"=w477) -> ("RobotDriveDevRef"=w473:T5)  [unwired: 1 in, 7 out]
          n143 = Wait (ms)(milliseconds to wait=u32 150) -> ()  [unwired: 1 out]
        }
        frame #23 {
          n144 = call-poly <vilib>:"WPI_RobotDriveArcadeDrive.vi"("Y axis value"=0.0, "X axis value"=0.0, "RobotDriveDevRef"=w480) -> ()  [unwired: 1 in, 8 out]
        }
      }
      n145 = call-poly <vilib>:"SD Write Value.vi"("Boolean"=TRUE, "Name"="DB/LED 3" ("refnum name")) -> ()  [unwired: 8 in, 2 out]
    }
  }
